vi "AutoScheduleNew.vi"() -> ()   [LabVIEW 2012]
uses:
  <vilib>/Utility/NIReport.llb/NI_report.lvclass
  <vilib>/addons/database/Auxilliary.llb/DB Tools Cursor Type.ctl
  <vilib>/addons/_office/_exclsub.llb/font.ctl
  <vilib>/addons/_office/excel.llb/Excel Get Data (str).vi
  <vilib>/addons/database/Connection.llb/DB Tools Open Connec (Path).vi
  <vilib>/addons/database/Connection.llb/Conn Execute.vi
  <vilib>/addons/database/Recordset.llb/Rec Fetch Recordset Data (R).vi
  <vilib>/addons/database/Recordset.llb/Rec Destroy - Connection.vi
  <vilib>/Utility/NIReport.llb/Excel/NI_Excel.lvclass
  <vilib>/addons/_office/NI_ReportGenerationToolkit.lvlib
  <vilib>/addons/database/NI_Database_API.lvlib
panel:
  out "error out":errorcluster
  out "concatenated string 2":string
  out "error out 5":errorcluster
  in  "start (0, 0) 4":cluster{"start row":i32, "start column":i32}
  out "concatenated string":string
  in  "start (0, 0) 3":cluster{"start row":i32, "start column":i32}
  out "Numeric":i32
  out "ExcelRow":i32
  in  "start (0, 0)":cluster{"start row":i32, "start column":i32}
  out "x+y":i32
  in  "start (0, 0) 2":cluster{"start row":i32, "start column":i32}
  out "row":i32
  out "array":string[][](array[string])
  out "error out 4":errorcluster
  out "spreadsheet string":string
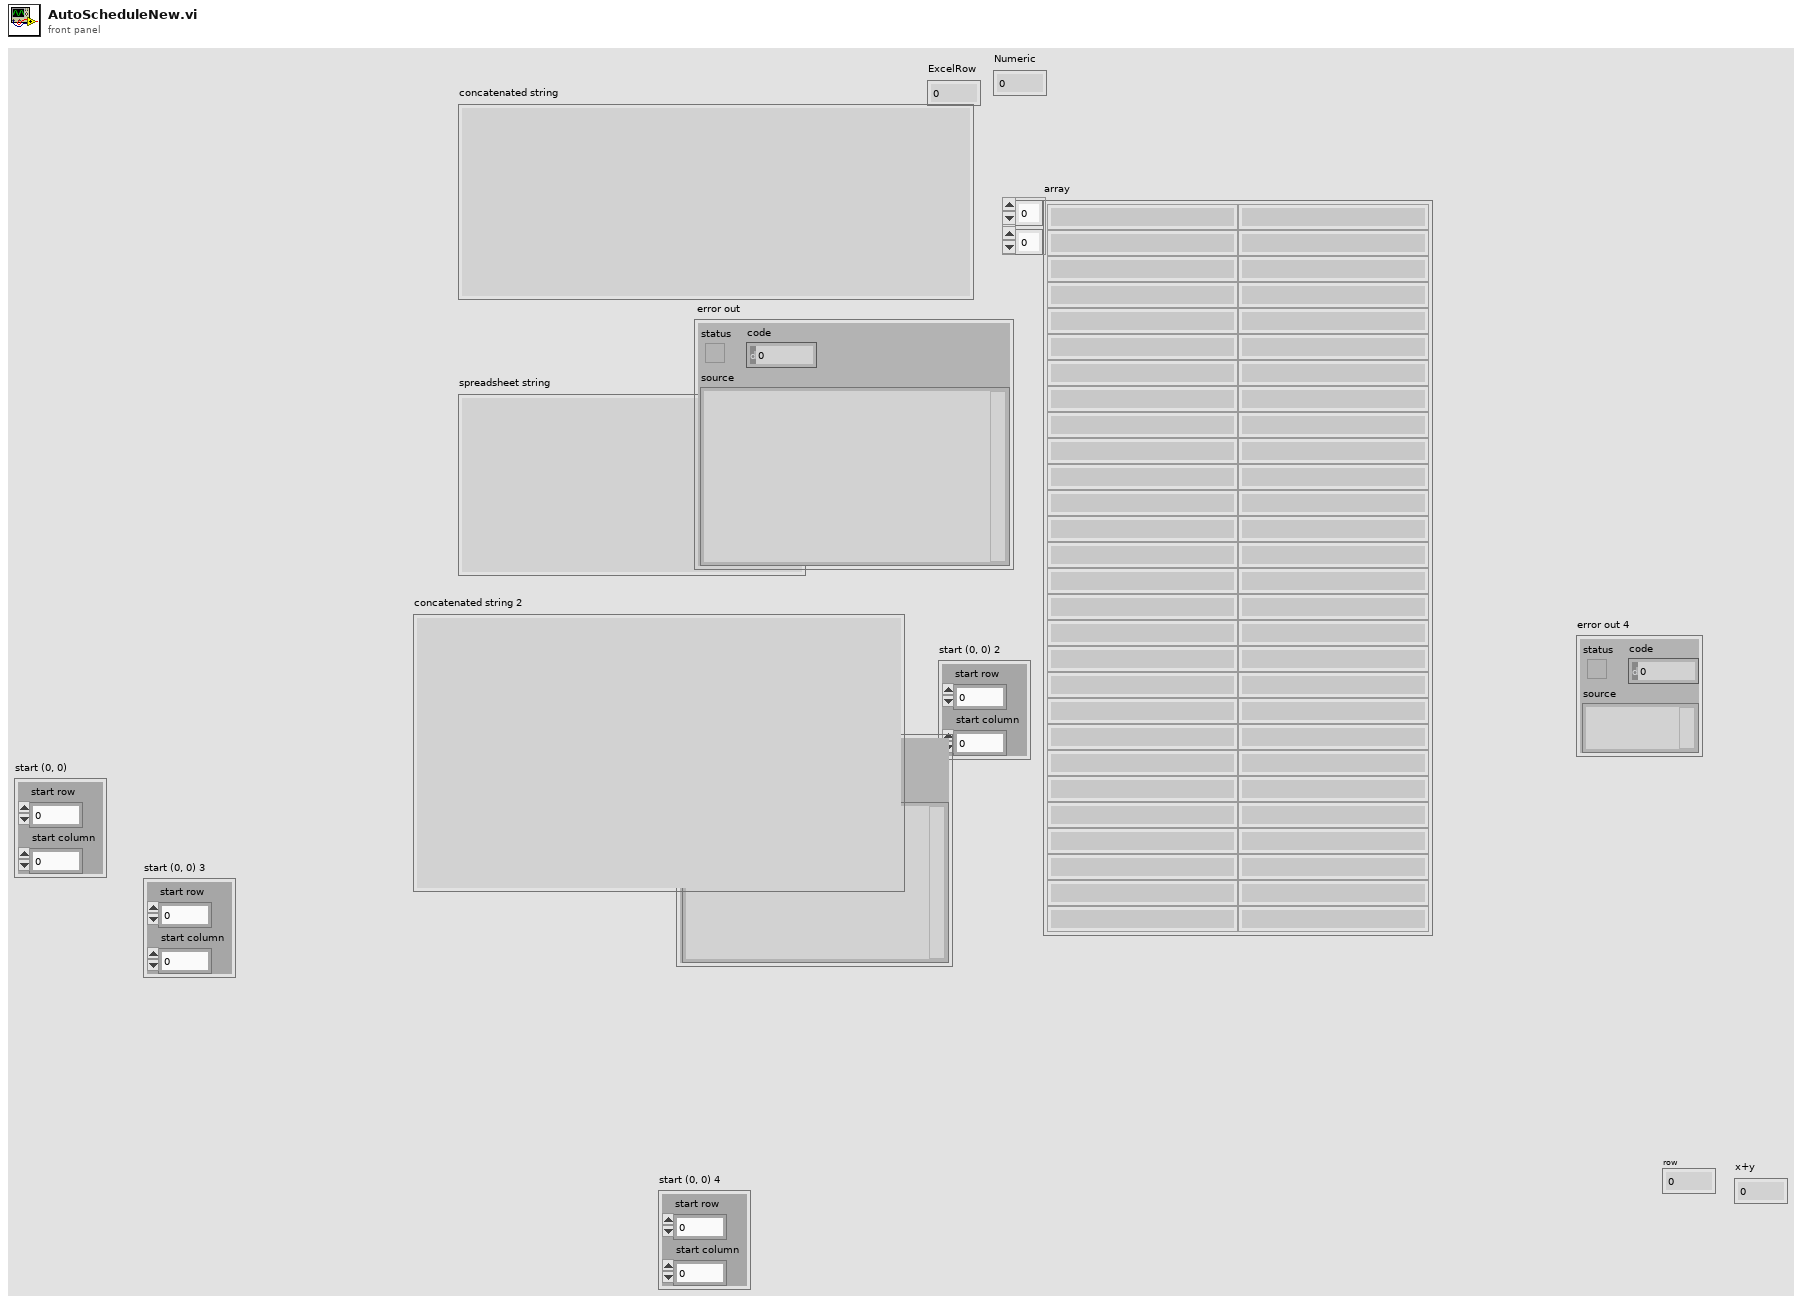
[diagram p1: front panel]
types:
  T1 = enum16{"Standard Report", "HTML", "Word", "Excel"}
  T2 = typedef "NI_ReportGenerationToolkit.lvlib/font.ctl" = cluster{"font name":string, "font size":dbl, "bold":u16, "italic":u16, "underline":u16, "strike through":u16, "font color":u32}
  T3 = cluster{"on/off":bool, "weight":i32, "color":u32}
  T4 = typedef "NI_Database_API.lvlib/DB Tools Cursor Type.ctl" = enum16{"forward-only", "keyset", "dynamic", "static"}
  T5 = typedef "NI_Database_API.lvlib/Conn ObjectReference.ctl" = refnum<k1>
  T6 = typedef "NI_Database_API.lvlib/Rec ObjectReference.ctl" = refnum<k1>
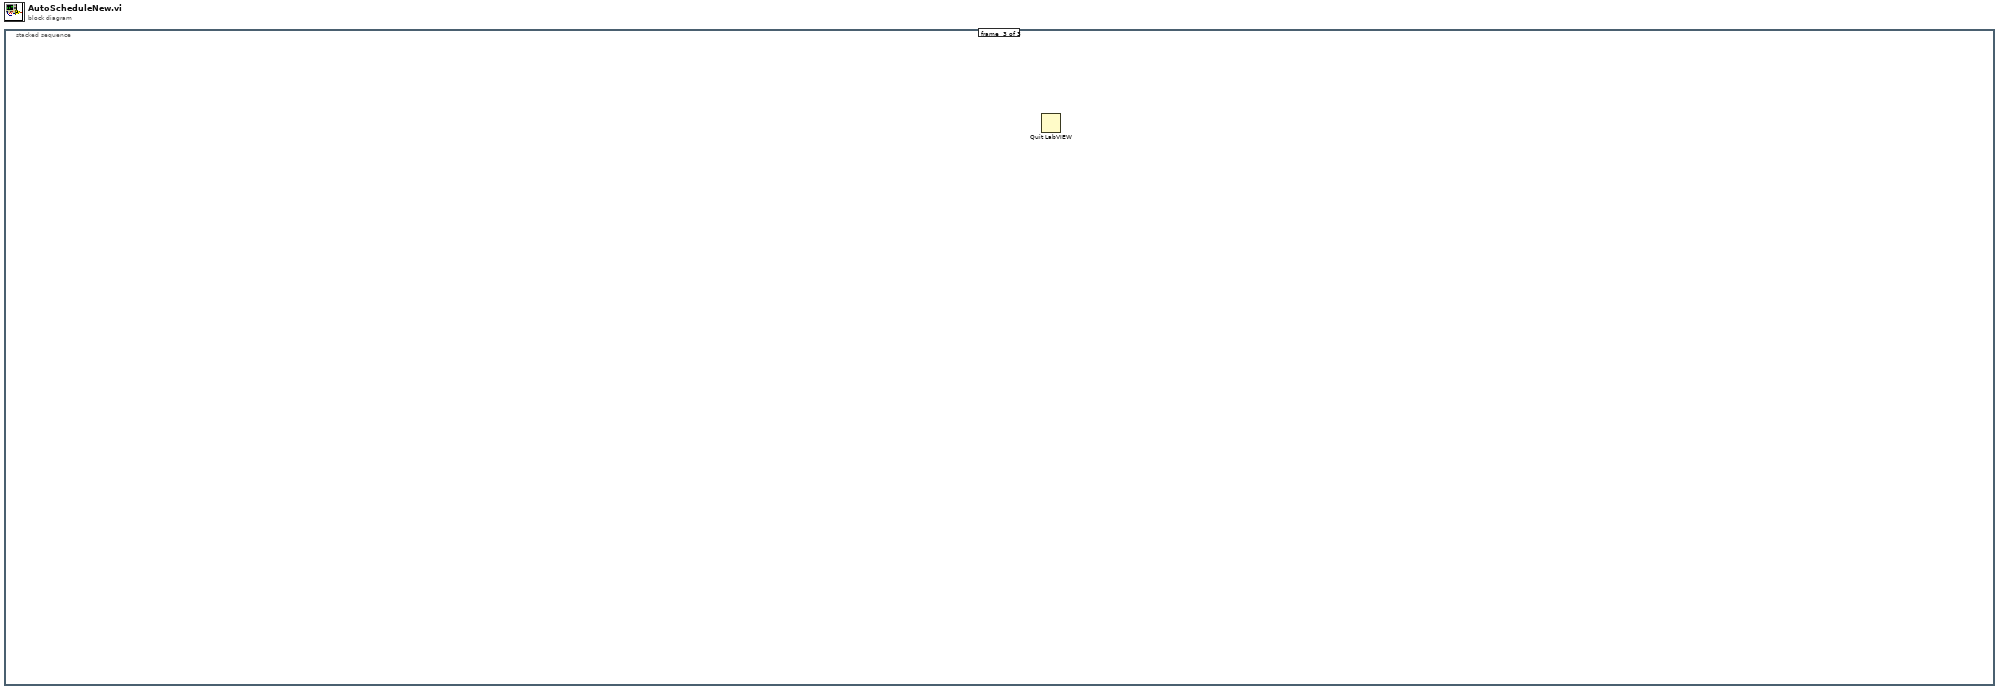
[diagram p0: block diagram]
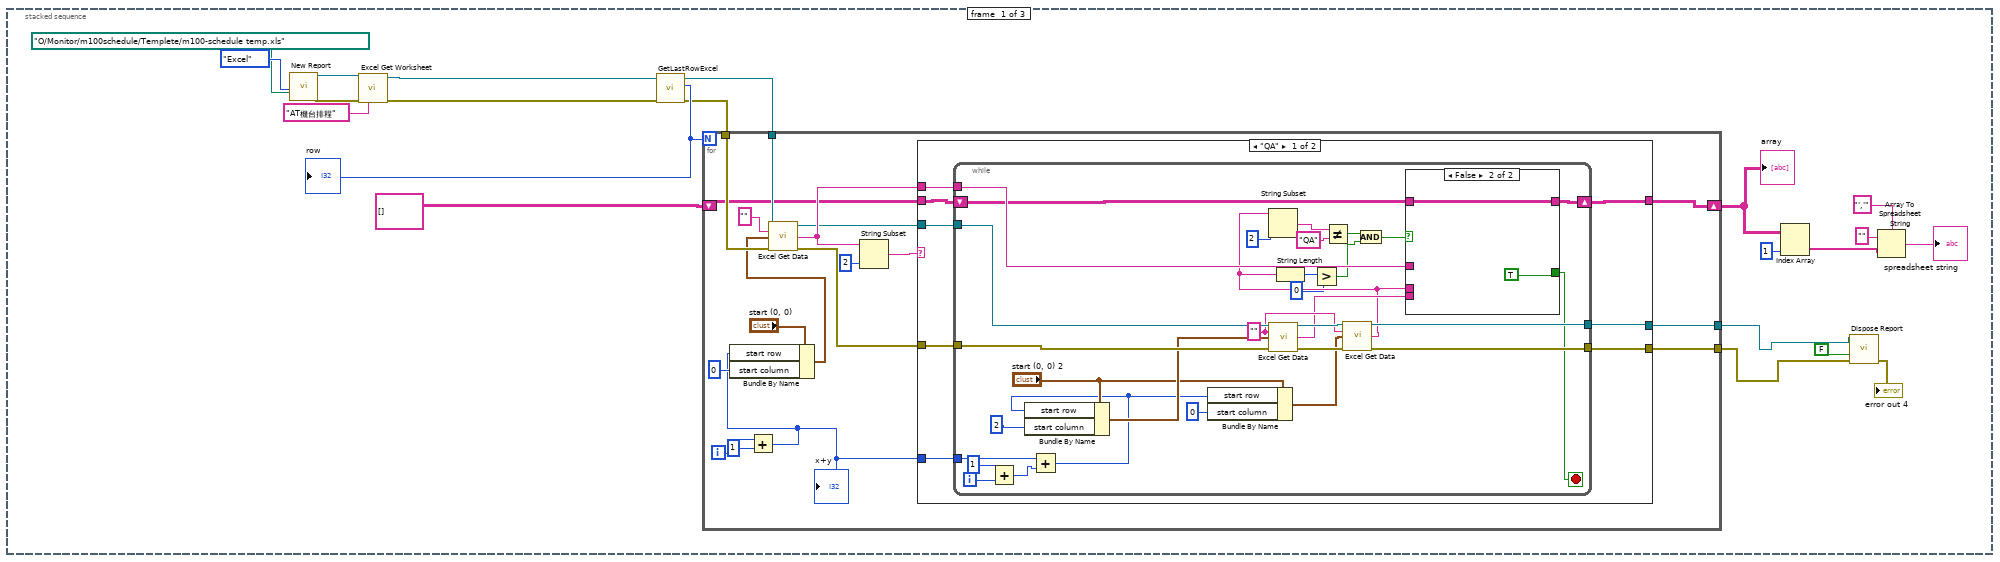
[diagram p2: hidden frame]
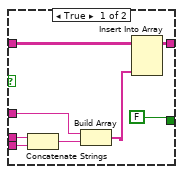
[diagram p3: hidden frame]
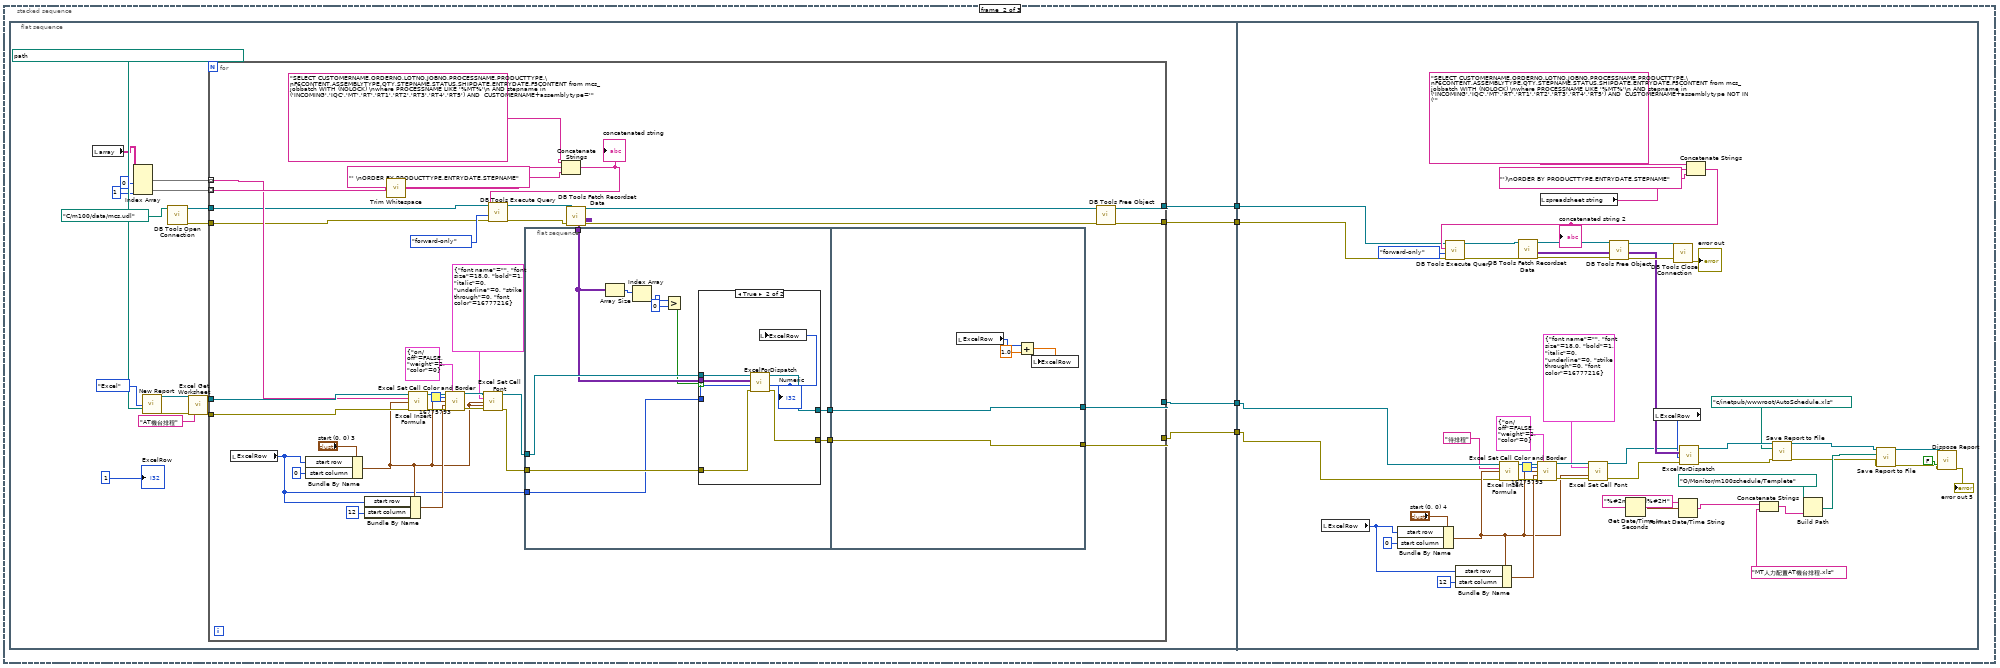
[diagram p5: hidden frame]
diagram:
  n1 = stacked-sequence {
    frame #0 {
      n2 = call <vilib>:"New Report.vi"("report type"=T1."Excel" ("Report Type"), "template (empty)"=path "O:/Monitor/m100schedule/Templete/m100-schedule temp.xls") -> ("report out"=w20:refnum<class "NI_report.lvclass">, "error out"=w19:errorcluster)  [unwired: 12 in]
      n3 = call <vilib>:"Excel Get Worksheet.vi"("report in"=w20, "error in (no error)"=w19, "name (\"\")"="AT機台排程" ("name (\"\")")) -> ("report out"=w18:refnum<class "NI_report.lvclass">, "error out"=w17:errorcluster)  [unwired: 11 in]
      n4 = call "GetLastRowExcel.vi"("error in (no error)"=w17, "report in"=w18) -> ("error out"=w13:errorcluster, "row"=w16:i32, "report out"=w12:refnum<class "NI_report.lvclass">)  [unwired: 7 in]
      "row" <- w16
      n5 = for {
        N: w16 -> [_]
        tunnel: w12 -> [w39]
        tunnel: w13 -> [w38]
        shift-right: [w27] -> w3
        shift-left: string[][] [] ("array") -> [w28]
        tunnel: [w23] -> w8
        tunnel: [w22] -> w7
        i -> [w34]
        n6 = Add(x=w34, y=1) -> (x+y=w24:i32)
        "x+y" <- w24
        n7 = Bundle By Name(cluster="start (0, 0)", "start row"=w24, "start column"=0) -> (w35:cluster{"start row":i32, "start column":i32})
        n8 = call-poly <vilib>:"Excel Get Data.vi"("report in"=w39, "data type"="", "start (0, 0)"=w35, "error in (no error)"=w38) -> ("report out"=w26:refnum<class "NI_report.lvclass">, "data"=w30:string, "error out"=w25:errorcluster)  [unwired: 9 in]
        n9 = String Subset(string=w30, length (rest)=2 ("length (rest)")) -> (substring=w31:string)  [unwired: 1 in]
        n10 = case shown="\"QA\"" w31 {
          tunnel: w30 -> [w47 _]
          tunnel: w28 -> [w40 w91]
          tunnel: [w46 w91] -> w27
          tunnel: w26 -> [w45 w90]
          tunnel: w25 -> [w44 w89]
          tunnel: w24 -> [w43 _]
          tunnel: [w42 w90] -> w23
          tunnel: [w41 w89] -> w22
          frame "QA" {
            n11 = while {
              tunnel: w47 -> [w78]
              tunnel: w45 -> [w77]
              tunnel: w44 -> [w76]
              tunnel: w43 -> [w73]
              tunnel: [w71] -> w42
              tunnel: [w69] -> w41
              shift-right: [w56] -> w46
              shift-left: w40 -> [w55]
              i -> [w62]
              stop <- w54 stop-if-true
              w68 = "" ("data type")
              n12 = Add(x=1, y=w62) -> (x+y=w60:i32)
              n13 = Add(x=w73, y=w60) -> (x+y=w65:i32)
              n14 = Bundle By Name(cluster="start (0, 0) 2", "start row"=w65, "start column"=2) -> (w75:cluster{"start row":i32, "start column":i32})
              n15 = Bundle By Name(cluster="start (0, 0) 2", "start row"=w65, "start column"=0) -> (w67:cluster{"start row":i32, "start column":i32})
              n16 = call-poly <vilib>:"Excel Get Data.vi"("report in"=w77, "data type"=w68, "start (0, 0)"=w75, "error in (no error)"=w76) -> ("report out"=w72:refnum<class "NI_report.lvclass">, "data"=w63:string, "error out"=w70:errorcluster)  [unwired: 9 in]
              n17 = call-poly <vilib>:"Excel Get Data.vi"("report in"=w72, "data type"=w68, "start (0, 0)"=w67, "error in (no error)"=w70) -> ("report out"=w71:refnum<class "NI_report.lvclass">, "data"=w53:string, "error out"=w69:errorcluster)  [unwired: 9 in]
              n18 = String Subset(string=w53, length (rest)=2 ("length (rest)")) -> (substring=w58:string)  [unwired: 1 in]
              n19 = String Length(string=w53) -> (length=w52:i32)
              n20 = Greater?(x=w52, y=0) -> (0:w49:bool)
              n21 = Not Equal?(x=w58, y="QA") -> (x != y?=w50:bool)
              n22 = And(x=w50, y=w49) -> (x .and. y?=w48:bool)
              n23 = case shown="False" w48 {
                tunnel: w78 -> [w86 _]
                tunnel: w55 -> [w83 w88]
                tunnel: w53 -> [w82 _]
                tunnel: w63 -> [w81 _]
                tunnel: [w84 w88] -> w56
                tunnel: [FALSE TRUE] -> w54
                frame True {
                  n24 = Concatenate Strings(w82, w81) -> (w80:string)
                  n25 = Build Array(w86, w80) -> (w85:string[])
                  n26 = Insert Into Array(array=w83, new element=w85) -> (w84:string[][])  [unwired: 2 in]
                }
                frame False {
                }
              }
            }
          }
          frame Default {
          }
        }
      }
      "array" <- w3
      n27 = Index Array(array=w3, index (col)=1 ("disabled index (col)")) -> (element=w1:string[])  [unwired: 1 in]
      n28 = call-dynamic "Dispose Report.vi"("report in"=w8, "save changes? (F)"=FALSE, "error in (no error)"=w7) -> ("error out"=→"error out 4":errorcluster)  [unwired: 12 in]
      n29 = Array To Spreadsheet String(delimiter (Tab)="','", array=w1, 3:"" ("format string")) -> (spreadsheet string=→"spreadsheet string":string)
    }
    frame #1 {
      n30 = flat-sequence {
        tunnel: [w99] -> w95
        tunnel: [w98] -> w94
        tunnel: [w97] -> w93
        tunnel: [w96] -> w92
        tunnel: w95 -> [w213]
        tunnel: w94 -> [w212]
        tunnel: w93 -> [w184]
        tunnel: w92 -> [w183]
        frame #0 {
          n31 = local read "array"() -> (w110:string[][])
          n32 = Index Array(array=w110, index (col) #1=0 ("disabled index (col)"), index (col) #2=1 ("index (col)")) -> (element #1=w109:string[], element #2=w106:string[])  [unwired: 2 in]
          n33 = call <vilib>:"New Report.vi"("report type"=T1."Excel" ("Report Type"), "template (empty)"=path "O:/Monitor/m100schedule/Templete/MT人力配置AT機台排程.xls" ("template (empty) 2")) -> ("report out"=w114:refnum<class "NI_report.lvclass">, "error out"=w113:errorcluster)  [unwired: 12 in]
          n34 = call-poly <vilib>:"DB Tools Open Connection.vi"("connection information"=path "C:/m100/data/mcs.udl") -> ("error out"=w100:errorcluster, "connection reference"=w101:T5)  [unwired: 7 in]
          n35 = call <vilib>:"Excel Get Worksheet.vi"("report in"=w114, "error in (no error)"=w113, "name (\"\")"="AT機台排程" ("name (\"\")")) -> ("report out"=w105:refnum<class "NI_report.lvclass">, "error out"=w104:errorcluster)  [unwired: 11 in]
          n36 = for {
            tunnel: w109 -> [w139] mode=indexing
            tunnel: w106 -> [w144] mode=indexing
            tunnel: w105 -> [w141]
            tunnel: w104 -> [w140]
            tunnel: [w124] -> w97
            tunnel: [w123] -> w96
            tunnel: w101 -> [w122]
            tunnel: w100 -> [w121]
            tunnel: [w120] -> w99
            tunnel: [w119] -> w98
            n37 = local read "ExcelRow"() -> (w116:i32)
            n38 = Bundle By Name(cluster="start (0, 0) 3", "start row"=w116, "start column"=0) -> (w126:cluster{"start row":i32, "start column":i32})
            n39 = Bundle By Name(cluster=w126, "start row"=w116, "start column"=12) -> (w131:cluster{"start row":i32, "start column":i32})
            n40 = call <vilib>:"Trim Whitespace.vi"("string"=w144) -> ("trimmed string"=w143:string)  [unwired: 1 in]
            n41 = call <vilib>:"Excel Insert Formula.vi"("report in"=w141, "formula"=w139, "start (0, 0)"=w126, "error in (no error)"=w140) -> ("report out"=w136:refnum<class "NI_report.lvclass">, "error out"=w135:errorcluster)  [unwired: 10 in]
            n42 = call <vilib>:"Excel Set Cell Color and Border.vi"("report in"=w136, "inside border"=T3 {"on/off"=FALSE, "weight"=2, "color"=0}, "background color (w)"=u32 16775793, "start (-1, -1)"=w126, "end (-1, -1)"=w131, "error in (no error)"=w135) -> ("report out"=w130:refnum<class "NI_report.lvclass">, "error out"=w129:errorcluster)  [unwired: 8 in]
            n43 = call <vilib>:"Excel Set Cell Font.vi"("report in"=w130, "font"=T2 {"font name"="", "font size"=18.0, "bold"=1, "italic"=0, "underline"=0, "strike through"=0, "font color"=16777216}, "start (-1, -1)"=w126, "end (-1, -1)"=w126, "error in (no error)"=w129) -> ("report out"=w128:refnum<class "NI_report.lvclass">, "error out"=w127:errorcluster)  [unwired: 9 in]
            n44 = flat-sequence {
              tunnel: w142 -> [w157]
              tunnel: w128 -> [w162]
              tunnel: w127 -> [w161]
              tunnel: [w160] -> w118
              tunnel: [w159] -> w117
              tunnel: w116 -> [w158]
              tunnel: [w173] -> w124
              tunnel: w118 -> [w173]
              tunnel: [w172] -> w123
              tunnel: w117 -> [w172]
              frame #0 {
                n45 = Array Size(array=w157) -> (size(s)=w156:i32[])
                n46 = Index Array(array=w156) -> (element=w155:i32)  [unwired: 1 in]
                n47 = Greater?(x=w155, y=0) -> (0:w153:bool)
                n48 = case shown="True" w153 {
                  tunnel: w162 -> [w164 w171]
                  tunnel: w161 -> [w163 w170]
                  tunnel: [w164 w169] -> w160
                  tunnel: [w163 w168] -> w159
                  tunnel: w158 -> [_ w166]
                  tunnel: w157 -> [_ w165]
                  frame False {
                  }
                  frame True {
                    n49 = call "ExcelForDispatch.vi"("error out"=w170, "RowNo"=w166, "array"=w165, "report out"=w171) -> ("error out 2"=w168:errorcluster, "Numeric"=w167:i32, "report out 2"=w169:refnum<class "NI_report.lvclass">)  [unwired: 5 in]
                    "Numeric" <- w167
                    n50 = local write "ExcelRow"(w167) -> ()
                  }
                }
              }
              frame #1 {
                n51 = local read "ExcelRow"() -> (w175:i32)
                n52 = Add(x=w175, y=1.0) -> (x+y=w174:dbl)
                n53 = local write "ExcelRow"(w174) -> ()
              }
            }
            n54 = Concatenate Strings("SELECT CUSTOMERNAME,ORDERNO,LOTNO,JOBNO,PROCESSNAME,PRODUCTTYPE,\nF6CONTENT,ASSEMBLYTYPE,QTY,STEPNAME,STATUS,SHIPDATE,ENTRYDATE,F5CONTENT from mcs_jobbatch WITH (NOLOCK) \nwhere PROCESSNAME LIKE '%MT%'\n AND stepname in ('INCOMING','IQC','MT','RT','RT1','RT2','RT3','RT4','RT5') AND  CUSTOMERNAME+assemblytype='" ("SQL query"), w143, "' \nORDER BY PRODUCTTYPE,ENTRYDATE,STEPNAME" ("string")) -> (w146:string)
            "concatenated string" <- w146
            n55 = call-poly <vilib>:"DB Tools Execute Query.vi"("error in (no error)"=w121, "cursor type"=DB_Tools_Cursor_Type."forward-only", "SQL query"=w146, "connection reference"=w122) -> ("error out"=w150:errorcluster, "recordset reference"=w152:T6)  [unwired: 4 in]
            n56 = call-poly <vilib>:"DB Tools Fetch Recordset Data.vi"("error in (no error)"=w150, "recordset reference"=w152) -> ("error out"=w149:errorcluster, "recordset data"=w142:variant[][], "recordset reference out"=w151:T6)  [unwired: 3 in]
            n57 = call-poly <vilib>:"DB Tools Free Object.vi"("error in (no error)"=w149, "recordset reference"=w151) -> ("error out"=w119:errorcluster, "connection reference"=w120:T5)  [unwired: 8 in]
          }
          "ExcelRow" <- 1
        }
        frame #1 {
          n58 = local read "ExcelRow"() -> (w187:i32)
          n59 = Bundle By Name(cluster="start (0, 0) 4", "start row"=w187, "start column"=0) -> (w189:cluster{"start row":i32, "start column":i32})
          n60 = Bundle By Name(cluster=w189, "start row"=w187, "start column"=12) -> (w192:cluster{"start row":i32, "start column":i32})
          n61 = call <vilib>:"Excel Insert Formula.vi"("report in"=w184, "formula"="待排程", "start (0, 0)"=w189, "error in (no error)"=w183) -> ("report out"=w197:refnum<class "NI_report.lvclass">, "error out"=w196:errorcluster)  [unwired: 10 in]
          n62 = call <vilib>:"Excel Set Cell Color and Border.vi"("report in"=w197, "inside border"=T3 {"on/off"=FALSE, "weight"=2, "color"=0}, "background color (w)"=u32 16775793, "start (-1, -1)"=w189, "end (-1, -1)"=w192, "error in (no error)"=w196) -> ("report out"=w191:refnum<class "NI_report.lvclass">, "error out"=w190:errorcluster)  [unwired: 8 in]
          n63 = local read "spreadsheet string"() -> (w218:string)
          n64 = call <vilib>:"Excel Set Cell Font.vi"("report in"=w191, "font"=T2 {"font name"="", "font size"=18.0, "bold"=1, "italic"=0, "underline"=0, "strike through"=0, "font color"=16777216}, "start (-1, -1)"=w189, "end (-1, -1)"=w189, "error in (no error)"=w190) -> ("report out"=w186:refnum<class "NI_report.lvclass">, "error out"=w185:errorcluster)  [unwired: 9 in]
          n65 = Get Date/Time In Seconds() -> (seconds since 1Jan1904=w202:timestamp)
          n66 = local read "ExcelRow"() -> (w214:i32)
          n67 = Format Date/Time String(time format string (%c)="%#2m%#2d%#2H", seconds (now)=w202) -> (date/time string=w200:string)  [unwired: 1 in]
          n68 = Concatenate Strings("SELECT CUSTOMERNAME,ORDERNO,LOTNO,JOBNO,PROCESSNAME,PRODUCTTYPE,\nF6CONTENT,ASSEMBLYTYPE,QTY,STEPNAME,STATUS,SHIPDATE,ENTRYDATE,F5CONTENT from mcs_jobbatch WITH (NOLOCK) \nwhere PROCESSNAME LIKE '%MT%'\n AND stepname in ('INCOMING','IQC','MT','RT','RT1','RT2','RT3','RT4','RT5') AND  CUSTOMERNAME+assemblytype NOT IN ('" ("SQL query"), w218, "')\nORDER BY PRODUCTTYPE,ENTRYDATE,STEPNAME" ("string")) -> (w216:string)
          "concatenated string 2" <- w216
          n69 = call-poly <vilib>:"DB Tools Execute Query.vi"("error in (no error)"=w212, "cursor type"=DB_Tools_Cursor_Type."forward-only", "SQL query"=w216, "connection reference"=w213) -> ("error out"=w224:errorcluster, "recordset reference"=w226:T6)  [unwired: 4 in]
          n70 = call-poly <vilib>:"DB Tools Fetch Recordset Data.vi"("error in (no error)"=w224, "recordset reference"=w226) -> ("error out"=w223:errorcluster, "recordset data"=w215:variant[][], "recordset reference out"=w225:T6)  [unwired: 3 in]
          n71 = call-poly <vilib>:"DB Tools Free Object.vi"("error in (no error)"=w223, "recordset reference"=w225) -> ("error out"=w222:errorcluster, "connection reference"=w221:T5)  [unwired: 8 in]
          n72 = call <vilib>:"DB Tools Close Connection.vi"("error in (no error)"=w222, "connection reference"=w221) -> ("error out"=→"error out":errorcluster)  [unwired: 5 in]
          n73 = call "ExcelForDispatch.vi"("error out"=w185, "RowNo"=w214, "array"=w215, "report out"=w186) -> ("error out 2"=w180:errorcluster, "report out 2"=w181:refnum<class "NI_report.lvclass">)  [unwired: 5 in, 1 out]
          n74 = Concatenate Strings(w200, "MT人力配置AT機台排程.xls" ("string")) -> (w204:string)
          n75 = call-dynamic "Save Report to File.vi"("report in"=w181, "report file path"=path "c:/inetpub/wwwroot/AutoSchedule.xls", "error in (no error)"=w180) -> ("report out"=w179:refnum<class "NI_report.lvclass">, "error out"=w178:errorcluster)  [unwired: 11 in]
          n76 = Build Path(base path=path "O:/Monitor/m100schedule/Templete", name or relative path=w204) -> (appended path=w205:path)
          n77 = call-dynamic "Save Report to File.vi"("report in"=w179, "report file path"=w205, "error in (no error)"=w178) -> ("report out"=w207:refnum<class "NI_report.lvclass">, "error out"=w206:errorcluster)  [unwired: 11 in]
          n78 = call-dynamic "Dispose Report.vi"("report in"=w207, "save changes? (F)"=FALSE, "error in (no error)"=w206) -> ("error out"=→"error out 5":errorcluster)  [unwired: 12 in]
        }
      }
    }
    frame #2 {
      n79 = Quit LabVIEW() -> ()  [unwired: 1 in]
    }
  }
